vi "数组.vi"() -> ()   [LabVIEW 2015]
panel:
  out "对应值":dbl
  in  "输入索引号":dbl
  out "降序排列":dbl[](array[numeric])
  out "升序排列":dbl[](array[numeric])
  out "数组大小":dbl
  out "最后元素":dbl
  out "Array":dbl[](array[numeric])
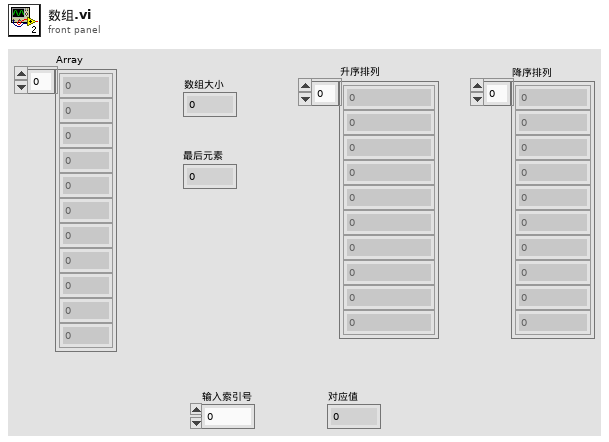
[diagram p1: front panel]
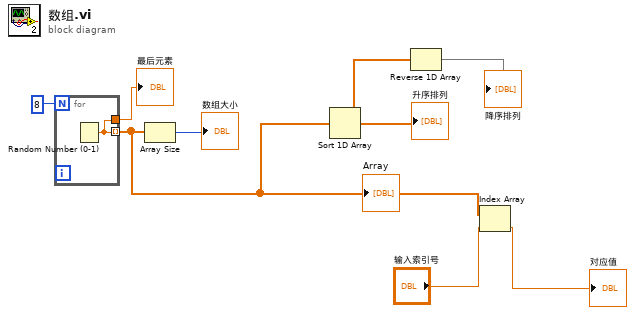
[diagram p0: block diagram]
diagram:
  n1 = for {
    N: 8 -> [_]
    tunnel: [w9] -> w7
    tunnel: [w9] -> w3 mode=indexing
    n2 = Random Number (0-1)() -> (number: 0 to 1=w9:dbl)
  }
  "Array" <- w3
  "最后元素" <- w7
  n3 = Array Size(array=w3) -> (size(s)=→"数组大小":i32)
  n4 = Sort 1D Array(array=w3) -> (sorted array=w5:dbl[])
  "升序排列" <- w5
  n5 = Reverse 1D Array(array=w5) -> (reversed array=→"降序排列":dbl[])
  n6 = Index Array(array=w3, index="输入索引号") -> (element=→"对应值":dbl)
